vi "Initialise ctrl values.vi"(8 "error in (no error)":errorcluster) -> (0 "error out":errorcluster)   [LabVIEW 2020]
uses:
  Typedefs/HW config states enum.ctl
  Typedefs/Read Write Enum.ctl
  Typedefs/AOL modes.ctl
  Global Variables/gl_UI Ctrl Refs.vi
  Peripherals Control/Pockels/Globals/gl_Pockels control globals.vi
  Global Variables/General Globals.vi
  Typedefs/Laser control knob.ctl
  Typedefs/PMT control knob.ctl
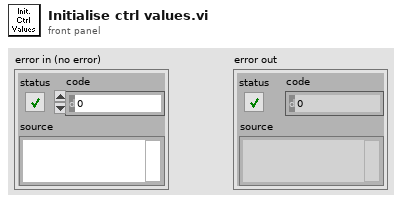
[diagram p1: front panel]
types:
  T1 = typedef "HW config states enum.ctl" = enum16{"Load from file", "Save to file", "Save backup", "Write all", "Read all", "Write XY stage settings", "Write DAQ FPGA settings", "Write Control FPGA settings", "Write Phys Channels", "Write System Config", "Write HW Config", "Save System Config", "Save HW Config", "Clear", "Compare from file"}
  T2 = typedef "UI ctrl refs cluster.ctl" = cluster{"Top level VI path":path, "Top level VI ref":refnum<vi>, "User menu ref":refnum<k9>, "Sub Panel control":refnum<vi>, "Imaging Param Tab":refnum<vi>, "Occurrence-Start drivers":refnum<k4>, "Occurrence-Speed logging initialised":refnum<k4>, "Occurrence-XYZ stage initialised":refnum<k4>, "Exit button":refnum<vi>, "Status ind":refnum<vi>, "Set as origin":refnum<vi>, "Speed Logging":refnum<vi>, "Time Lapse":refnum<vi>, "Live Imaging":refnum<vi>, "AOL Z Stack":refnum<vi>, "Motor Z Stack":refnum<vi>, "Funct Acq button":refnum<vi>, "Hard Shutter":refnum<vi>, "Virtual Shutter":refnum<vi>, "Laser Power":refnum<vi>, "AOL Mode":refnum<vi>, "Frame Size":refnum<vi>, "Field of View":refnum<vi>, "Dwell Time":refnum<vi>, "Zoom":refnum<vi>, "AOL Z":refnum<vi>, "Objective":refnum<vi>, "Axis":refnum<vi>, "Paths & Names":refnum<vi>, "Experiment folder path (ind.)":refnum<vi>, "Last State (Ind.)":refnum<vi>, "Averages":refnum<vi>, "Angle (degrees)":refnum<vi>, "X centre":refnum<vi>, "Y centre":refnum<vi>, "Plane Mode":refnum<vi>, "# Planes":refnum<vi>, "Z Start":refnum<vi>, "Z Stop":refnum<vi>, "Z Step":refnum<vi>, "PMT 1":refnum<vi>, "PMT 2":refnum<vi>, "Stage XYZ Position":refnum<vi>, "Pockels@Z Start":refnum<vi>, "Pockels@Z Stop":refnum<vi>, "Obtain Z Start":refnum<vi>, "Obtain Z Stop":refnum<vi>, "Live stim.trig.period":refnum<vi>, "Live stim.trig.enable":refnum<vi>, "Movement Correction":refnum<vi>, "Load Reference Image":refnum<vi>, "XY Stage Move":refnum<vi>, "MovCor Cluster":refnum<vi>, "RefDAQParam":refnum<vi>, "Funct. Acq. Pockels Modulation":refnum<vi>, "Ref Laser Power":refnum<vi>, "Enable Video Recording":refnum<vi>, "Video Record-Live Imaging":refnum<vi>, "Video Record-Funct acq":refnum<vi>, "Reference Source":refnum<vi>, "AOL Z-stack Chirps Ready (ind)":refnum<vi>, "Target time between mov.cor. ref triggers (ms)":refnum<vi>, "Funct. Acq. Ref frame save":refnum<vi>, "Tracking button":refnum<vi>, "Show ref plots window":refnum<vi>, "Center freq ind (nm)":refnum<vi>, "Pickup mode (ind)":refnum<vi>, "Logging queue (ind)":refnum<vi>, "Back aperture power (ind.)":refnum<vi>, "Power after objective (ind.)":refnum<vi>, "Switch user":refnum<vi>, "Ls1 Conn. Status":refnum<vi>, "Ls1Tuning Status":refnum<vi>, "Ls1 Faults":refnum<vi>, "Ls1 Connection":refnum<vi>, "Ls1 Mode":refnum<vi>, "Ls1 POWER [mW]":refnum<vi>, "Ls1Shutter":refnum<vi>, "Ls1 Wavelength":refnum<vi>, "Ls1 Note":refnum<vi>, "Ls1 Confirm Wav":refnum<vi>, "Ls1 PreChrp Prism1":refnum<vi>, "Ls1 PreChrp Prism2":refnum<vi>, "Ls1 wav top Ind":refnum<vi>, "Ls1 power top Ind":refnum<vi>, "Ls1 Pump peak Hold":refnum<vi>, "Ls1 Status Ind":refnum<vi>, "Ls1 wav cancel":refnum<vi>, "Experiment Type":refnum<vi>, "Biology Information":refnum<vi>, "Camera recording status":refnum<vi>}
  T3 = typedef "System Configuration.ctl" = cluster{"Laser wavelength (nm)":dbl, "DAQ FPGA System":T4, "Control system":T5}
  T4 = typedef "DAQ FPGA system config.ctl" = cluster{"Clock Freq (MHz) ":dbl, "Samples Wait after Trigger":u16, "AOD fill":u16, "StartupDelay":i32, "Slip Cycle (clock cycles)":u32, "Add Cycle":bool}
  T5 = typedef "CTRL system config.ctl" = cluster{"AOD 1 Amplitude":i16, "AOD 2 Amplitude":i16, "AOD 3 Amplitude":i16, "AOD 4 Amplitude":i16, "AOD 5 Amplitude":i16, "AOD 6 Amplitude":i16, "T0 (ns)":dbl, "Ta (ns)":dbl, "Data Time Interval (ns)":dbl, "Ctrl FPGA Clock (MHz)":dbl}
  T6 = typedef "AOL_Globals.ctl" = cluster{"Imaging Protocol":T7, "Number of POI":u16, "Number of Miniscans":u16, "Number of Trials":u16, "Number of Cycles ":u64, "# Averaged Frames":u16, "Laser power (%)":u8, "Pockels (V)":dbl, "Acquisition Length (sec)":dbl, "Fill time (us)":dbl, "POI Dwell time (us)":dbl, "Miniscan Dwell time per pixel (us)":dbl, "PMT 1":dbl, "PMT 2":dbl, "Back Apperture (mA)":dbl, "Frame Size":T8, "Center Frequency":dbl, "Field of View (norm)":dbl, "DwellTime (us)":dbl, "Wavelength (nm)":dbl, "Zoom":dbl, "AOL Z":dbl, "AOL Mode":T9, "GridXY":dbl, "GridZ":dbl, "TriggerPeriod (sec)":dbl, "Number of Pixels in Miniscan":u16, "Experiment folder path":path, "X centre":dbl, "Y centre":dbl, "Angle (degrees)":dbl, "Plane Mode":T10, "Threshold":u16[], "Regenerate Chirps":bool, "Rectangle ROI length (pixels)":u16, "Rectangle ROI height (pixels)":u16, "AOD fill":u16, "StartupDelay":i32, "Samples Wait after Trigger":u16, "Slip Cycle":u32, "Add Cycle":bool, "Functional Mode":T11, "Z Start":dbl, "Z Stop":dbl, "# Planes":i32, "Total Pixels":i32, "Variable Miniscan Pixels":u16[], "Use Variable Length":bool, "Use Variable Resolution":bool, "Laser power (%) at Z Start":u8, "Laser power (%) at Z Stop":u8, "Ref Z Step":i8, "Ref Dwell Time (us)":dbl, "Field of View (um)":dbl}
  T7 = typedef "Imaging Protocols enum.ctl" = enum16{"AOL Z-Stack", "Motor Z Stack", "Functional Acquisition", "Single Plane Acquisition", "Volume Acquisition", "Live Imaging", "Live Plane Imaging", "Live Volume Imaging"}
  T8 = typedef "Frame Size.ctl" = u16
  T9 = typedef "AOL modes.ctl" = enum16{"Raster", "Structural", "Pointing", "Mini Scan", "Alignment"}
  T10 = typedef "Plane Mode.ctl" = u16
  T11 = typedef "Functional Mode.ctl" = enum16{"Point", "Line", "Patch", "Plane", "Volume"}
  T12 = enum8{"Enabled", "Disabled", "Disabled and Grayed Out"}
  T13 = typedef "Laser control knob.ctl" = u16
  T14 = typedef "Read Write Enum.ctl" = enum16{"Read", "Write"}
  T15 = typedef "Ref DAQ Param.ctl" = cluster{"Full Frame Size":u16, "Ref Field of View":sgl, "Ref Zoom":i8, "Ref_dwellTime":sgl, "Ref X-pixels-per-line(Npxr)":i16, "Ref Y-lines-per-image(Npyr)":i16, "Ref Z-lines-per-image":i16, "Ignore Z lines":i16, "Ref Scan Cycles":i32, "Ref threshold XY":u16, "Ref threshold Z":u16, "Ref average XY":u16, "Ref Average  Z":u16, "Proportional_scale":fxp<+,16,2>, "Integral_scale":fxp<+/-,16,12>, "Proportional_scale Z":fxp<+,16,2>, "Integral_scale Z":fxp<+/-,16,12>, "Diff_threshold":fxp<+,16,2>, "Diff_threshold _z":fxp<+,16,2>, "Sliding Average":bool, "Ref count reset enabled":bool}
  T16 = typedef "Control algorithm.ctl" = enum16{"PID", "Kalman"}
  T17 = typedef "PMT control knob.ctl" = u16
  T18 = typedef "test_fpga_control.ctl" = cluster{"x_offset_host":fxp<+/-,16,8>, "y_offset_host":fxp<+/-,16,8>, "use host offset":bool, "Set_Ref_Centroid":bool, "OldChirpCode":bool, "use array of offsets":bool, "x_offset_host array":fxp<+/-,16,8>[], "y_offset_host array ":fxp<+/-,16,8>[], "use host offset Z":bool, "swap Z":bool, "z_offset_host ":fxp<+/-,16,8>}
  T19 = typedef "Hardware Configuration settings.ctl" = cluster{"Dev. PC":bool, "Swap XY on stage":bool, "No of AOD":u8, "MC Supported":bool, "Axial MC":bool, "Computer MAC address":string, "Externalise Triggers":bool, "Trigger HW config":T20, "DAQmx Chan":T21, "XY stage available":bool, "XY Stage":T22, "Z stage available":bool, "Z Stage config cluster":T23, "Encoder available":bool, "Encoder":T24, "VidRec available":bool, "Cam VidRec":T25, "Laser Power Control HW config":T26, "Laser 1 available":bool, "Laser 1 config cluster":T27, "Prechirper 1 available":bool, "Prechirper 1 config cluster":T28, "Control system.FPGA available?":bool, "Control Sys. HW config":T29, "DAQ FPGA HW Config":T30, "PMT Voltage Range":T34}
  T20 = typedef "Triggers HW config.ctl" = cluster{"Available Device List":i32, "Device Address":string}
  T21 = typedef "DAQmx physical channels cluster.ctl" = cluster{"Pockels AO":tag, "Hard shutter AO":tag, "PMT AOs":tag, "Galvo AOs":tag, "Power meter AI":tag}
  T22 = typedef "XY Stage config cluster.ctl" = cluster{"COM port":refnum<visa-resource-name>, "Baudrate":i32, "Type":string}
  T23 = typedef "Z Stage config cluster.ctl" = cluster{"COM port":refnum<visa-resource-name>, "Baudrate":i32, "Type":string}
  T24 = typedef "Encoder config cluster.ctl" = cluster{"IP address":string, "Port":u16, "Wheel radius (cm)":dbl, "Encoder Trigger":tag}
  T25 = typedef "Cam VidRec HW config setup cluster.ctl" = cluster{"DO flag-Video record":tag, "DO flag-Trial start":tag}
  T26 = typedef "Laser Power Control HW config.ctl" = cluster{"Laser Power Control":string, "Laser Power Modulation Control":enum16{"NI", "FPGA"}}
  T27 = typedef "Laser 1 config cluster.ctl" = cluster{"COM port":refnum<visa-resource-name>, "Baud Rate":i32, "Type":string}
  T28 = typedef "PreChirper 1 config cluster.ctl" = cluster{"Type":string, "Baud Rate":i32, "COM port":refnum<visa-resource-name>}
  T29 = typedef "Control Sys HW config cluster.ctl" = cluster{"Control system.FPGA Type":enum16{"Virtex 5", "Virtex 7"}, "Control system.Network adapter name":string, "Control system.MAC address":string, "Control system.Ethernet Port":u32, "Control system.Ethernet Port Opened":bool}
  T30 = typedef "DAQ FPGA HW config cluster.ctl" = cluster{"FGPA Ref":T31, "Target":T32, "input card type":T33}
  T31 = typedef "FPGA Ref.ctl" = refnum<k20>
  T32 = typedef "nirio_resource_hc.ctl" = tag
  T33 = typedef "FPGA input type AC-DC.ctl" = enum16{"AC Card", "DC Card"}
  T34 = typedef "PMT Voltage Range.ctl" = cluster{"PMT Voltage Lower Limit":dbl, "PMT Voltage Upper Limit":dbl}
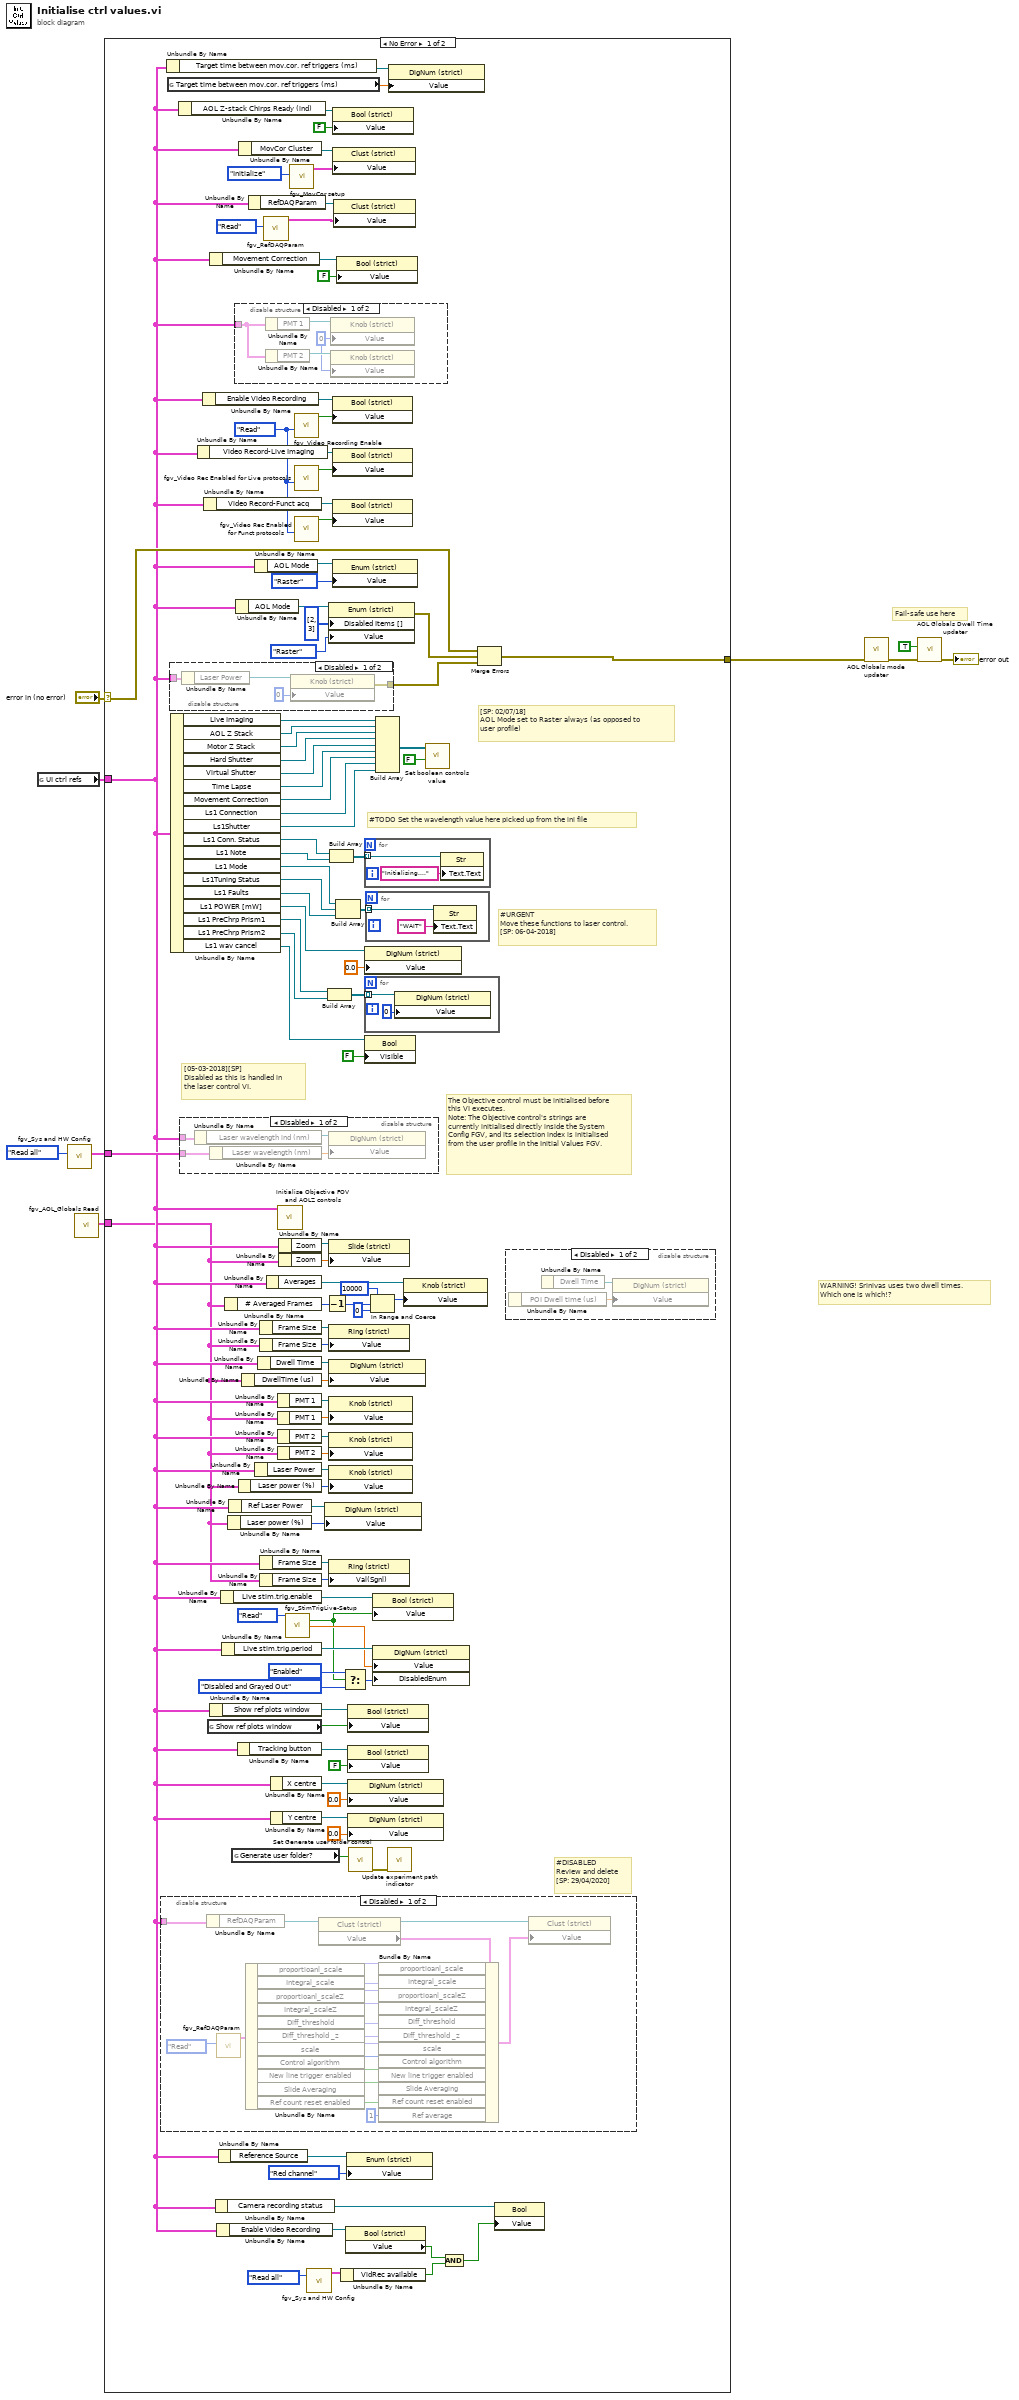
[diagram p0: block diagram]
diagram:
  # "Fail-safe use here"
  # "WARNING! Srinivas uses two dwell times.\nWhich one is which!?"
  n1 = global read "gl_UI Ctrl Refs.vi" "UI ctrl refs"() -> (w8:T2)
  n2 = call "fgv_Sys and HW Config.vi"("Function"=HW_config_states_enum."Read all") -> ("System Config OUT"=w1:T3)  [unwired: 8 in, 2 out]
  n3 = call "fgv_AOL_Globals Read.vi"() -> ("AOL_Globals"=w6:T6)  [unwired: 9 in, 2 out]
  n4 = case shown="No Error" "error in (no error)" {
    selector: "error in (no error)" -> [w45 w154]
    tunnel: w8 -> [w11 _]
    tunnel: [w102 w154] -> w5
    tunnel: w6 -> [w10 _]
    tunnel: w1 -> [w53 _]
    frame No Error {
      w96 = Read_Write_Enum."Read" ("Function")
      # "#DISABLED\nReview and delete\n[SP: 29/04/2020]"
      # "[SP: 02/07/18]\nAOL Mode set to Raster always (as opposed to \nuser profile)"
      # "#URGENT \nMove these functions to laser control.\n[SP: 06-04-2018]"
      # "[05-03-2018][SP]\nDisabled as this is handled in \nthe laser control VI."
      # "#TODO Set the wavelength value here picked up from the ini file"
      # "The Objective control must be initialised before this VI executes.\nNote: The Objective control's strings are currently initialised directly inside the System Config FGV, and its selection index is initialised from the user profile in the Initial Values FGV."
      n5 = disable-structure shown="Disabled" {
        disable-tunnel: w11 -> [w115 _]
        frame Disabled {
          n6 = Unbundle By Name(w115) -> ("RefDAQParam"=w133:refnum<vi>)
          n7 = call "fgv_RefDAQParam.vi"("Function"=enum16{"Initialize", "Write", "Read"}."Read") -> ("RefDAQParam"=w129:T15)  [unwired: 9 in, 1 out]
          n8 = Unbundle By Name(w129) -> ("proportioanl_scale"=w128:fxp<+,16,2>, "Integral_scale"=w127:fxp<+/-,16,12>, "proportioanl_scaleZ"=w126:fxp<+,16,2>, "Integral_scaleZ"=w125:fxp<+/-,16,12>, "Diff_threshold"=w124:fxp<+,16,2>, "Diff_threshold _z"=w123:fxp<+,16,2>, "scale"=w122:fxp<+,16,2>, "Control algorithm"=w121:T16, "New line trigger enabled"=w120:bool, "Slide Averaging"=w119:bool, "Ref count reset enabled"=w118:bool)
          n9 = property class="Clust (strict)"(reference=w133) -> (reference out=w117:refnum<vi>, "Value"=w132:T15)  [unwired: 1 in, 1 out]
          n10 = Bundle By Name(cluster=w132, "proportioanl_scale"=w128, "Integral_scale"=w127, "proportioanl_scaleZ"=w126, "Integral_scaleZ"=w125, "Diff_threshold"=w124, "Diff_threshold _z"=w123, "scale"=w122, "Control algorithm"=w121, "New line trigger enabled"=w120, "Slide Averaging"=w119, "Ref count reset enabled"=w118, "Ref average"=u16 1) -> (w131:T15)
          n11 = property class="Clust (strict)"(reference=w117, "Value"=w131) -> ()  [unwired: 1 in, 2 out]
        }
        frame Enabled {
        }
      }
      n12 = Unbundle By Name(w11) -> ("Target time between mov.cor. ref triggers (ms)"=w83:refnum<vi>)
      n13 = global read "gl_Pockels control globals.vi" "Target time between mov.cor. ref triggers (ms)"() -> (w82:dbl)
      n14 = disable-structure shown="Disabled" {
        disable-tunnel: [w147 _] -> w103
        disable-tunnel: w11 -> [w146 _]
        frame Disabled {
          n15 = Unbundle By Name(w146) -> ("Laser Power"=w149:refnum<vi>)
          n16 = property class="Knob (strict)"(reference=w149, "Value"=T13 0) -> (error out=w147:errorcluster)  [unwired: 1 in, 1 out]
        }
        frame Enabled {
        }
      }
      n17 = Unbundle By Name(w11) -> ("Live Imaging"=w114:refnum<vi>, "AOL Z Stack"=w113:refnum<vi>, "Motor Z Stack"=w112:refnum<vi>, "Hard Shutter"=w111:refnum<vi>, "Virtual Shutter"=w110:refnum<vi>, "Time Lapse"=w107:refnum<vi>, "Movement Correction"=w101:refnum<vi>, "Ls1 Connection"=w43:refnum<vi>, "Ls1Shutter"=w42:refnum<vi>, "Ls1 Conn. Status"=w41:refnum<vi>, "Ls1 Note"=w40:refnum<vi>, "Ls1 Mode"=w37:refnum<vi>, "Ls1Tuning Status"=w36:refnum<vi>, "Ls1 Faults"=w35:refnum<vi>, "Ls1 POWER [mW]"=w34:refnum<vi>, "Ls1 PreChrp Prism1"=w32:refnum<vi>, "Ls1 PreChrp Prism2"=w31:refnum<vi>, "Ls1 wav cancel"=w28:refnum<vi>)
      n18 = Unbundle By Name(w11) -> ("AOL Z-stack Chirps Ready (ind)"=w85:refnum<vi>)
      n19 = disable-structure shown="Disabled" {
        disable-tunnel: w53 -> [w135 _]
        disable-tunnel: w11 -> [w134 _]
        frame Disabled {
          n20 = Unbundle By Name(w134) -> ("Laser wavelength ind (nm)"=w137:refnum<vi>)
          n21 = Unbundle By Name(w135) -> ("Laser wavelength (nm)"=w136:dbl)
          n22 = property on="Property Node" class="DigNum (strict)"(reference=w137, "Value"=w136) -> ()  [unwired: 1 in, 2 out]
        }
        frame Enabled {
        }
      }
      n23 = Unbundle By Name(w11) -> ("Video Record-Live Imaging"=w95:refnum<vi>)
      n24 = Unbundle By Name(w11) -> ("Enable Video Recording"=w98:refnum<vi>)
      n25 = Unbundle By Name(w11) -> ("Video Record-Funct acq"=w94:refnum<vi>)
      n26 = global read "General Globals.vi" "Show ref plots window"() -> (w54:bool)
      n27 = Unbundle By Name(w11) -> ("Movement Correction"=w22:refnum<vi>)
      n28 = Unbundle By Name(w11) -> ("Show ref plots window"=w55:refnum<vi>)
      n29 = Unbundle By Name(w11) -> ("Camera recording status"=w15:refnum<vi>)
      n30 = Unbundle By Name(w11) -> ("Enable Video Recording"=w19:refnum<vi>)
      n31 = Unbundle By Name(w11) -> ("Reference Source"=w24:refnum<vi>)
      n32 = Unbundle By Name(w11) -> ("Live stim.trig.enable"=w62:refnum<vi>)
      n33 = Unbundle By Name(w11) -> ("Live stim.trig.period"=w61:refnum<vi>)
      n34 = Unbundle By Name(w10) -> ("# Averaged Frames"=w79:u16)
      n35 = Unbundle By Name(w10) -> ("Laser power (%)"=w13:u8)
      n36 = Unbundle By Name(w11) -> ("Ref Laser Power"=w12:refnum<vi>)
      n37 = global read "General Globals.vi" "Generate user folder?"() -> (w44:bool)
      n38 = disable-structure shown="Disabled" {
        disable-tunnel: w11 -> [w151 _]
        frame Disabled {
          w150 = T17 0 ("Value")
          n39 = Unbundle By Name(w151) -> ("PMT 1"=w153:refnum<vi>)
          n40 = Unbundle By Name(w151) -> ("PMT 2"=w152:refnum<vi>)
          n41 = property on="Property Node" class="Knob (strict)"(reference=w153, "Value"=w150) -> ()  [unwired: 1 in, 2 out]
          n42 = property on="Property Node" class="Knob (strict)"(reference=w152, "Value"=w150) -> ()  [unwired: 1 in, 2 out]
        }
        frame Enabled {
        }
      }
      n43 = Unbundle By Name(w11) -> ("AOL Mode"=w105:refnum<vi>)
      n44 = Unbundle By Name(w11) -> ("Tracking button"=w52:refnum<vi>)
      n45 = Unbundle By Name(w10) -> ("Laser power (%)"=w64:u8)
      n46 = Unbundle By Name(w11) -> ("MovCor Cluster"=w86:refnum<vi>)
      n47 = Unbundle By Name(w10) -> ("DwellTime (us)"=w70:dbl)
      n48 = Unbundle By Name(w11) -> ("RefDAQParam"=w89:refnum<vi>)
      n49 = Unbundle By Name(w11) -> ("AOL Mode"=w100:refnum<vi>)
      n50 = Unbundle By Name(w11) -> ("Laser Power"=w65:refnum<vi>)
      n51 = Unbundle By Name(w11) -> ("Dwell Time"=w71:refnum<vi>)
      n52 = Unbundle By Name(w11) -> ("Frame Size"=w72:refnum<vi>)
      n53 = Unbundle By Name(w10) -> ("Frame Size"=w73:T8)
      n54 = Unbundle By Name(w11) -> ("Frame Size"=w91:refnum<vi>)
      n55 = Unbundle By Name(w10) -> ("Frame Size"=w63:T8)
      n56 = call "fgv_RefDAQParam.vi"("Function"=enum16{"Initialize", "Write", "Read"}."Read" ("Status")) -> ("RefDAQParam"=w90:T15)  [unwired: 9 in, 1 out]
      n57 = Unbundle By Name(w11) -> ("Averages"=w78:refnum<vi>)
      n58 = Unbundle By Name(w11) -> ("X centre"=w50:refnum<vi>)
      n59 = Unbundle By Name(w11) -> ("Y centre"=w49:refnum<vi>)
      n60 = Unbundle By Name(w11) -> ("PMT 1"=w68:refnum<vi>)
      n61 = Unbundle By Name(w10) -> ("PMT 1"=w67:dbl)
      n62 = Unbundle By Name(w11) -> ("PMT 2"=w69:refnum<vi>)
      n63 = Unbundle By Name(w10) -> ("PMT 2"=w66:dbl)
      n64 = call "Initialise Objective FOV and AOLZ controls.vi"("UI ctrl refs"=w11) -> ()  [unwired: 10 in, 1 out]
      n65 = Unbundle By Name(w11) -> ("Zoom"=w81:refnum<vi>)
      n66 = Unbundle By Name(w10) -> ("Zoom"=w80:dbl)
      n67 = call "fgv_StimTrigLive-Setup.vi"("Function"=enum16{"Intialize", "Write", "Read", "Clear"}."Read") -> ("Live stim.trig.enable"=w46:bool, "Live stim.trig.period (sec)"=w59:dbl)  [unwired: 11 in, 2 out]
      n68 = call "fgv_MovCor setup.vi"("Status"=enum16{"Initialize", "Write", "Read"}."Initialize") -> ("MovCor Cluster"=w29:T18)  [unwired: 9 in, 1 out]
      n69 = call "fgv_Video Recording Enable.vi"("Function"=w96) -> ("Video Recording Enabled"=w97:bool)  [unwired: 9 in, 1 out]
      n70 = call "fgv_Video Rec Enabled for Live protocols.vi"("Function"=w96) -> ("Video Recording Enabled for Live protocols"=w92:bool)  [unwired: 10 in]
      n71 = call "fgv_Video Rec Enabled for Funct protocols.vi"("Function"=w96) -> ("Video Recording Enabled for functional acq protocols"=w93:bool)  [unwired: 10 in]
      n72 = call "fgv_Sys and HW Config.vi"("Function"=HW_config_states_enum."Read all") -> ("Hardware Configuration OUT"=w18:T19)  [unwired: 8 in, 2 out]
      n73 = Decrement(x=w79) -> (x-1=w77:u16)
      n74 = property class="DigNum (strict)"(reference=w12, "Value"=w13) -> ()  [unwired: 1 in, 2 out]
      n75 = Build Array(w32, w31) -> (w30:refnum<vi>[])
      n76 = property on="Property Node" class="Enum (strict)"(reference=w105, "Disabled Items []"=i32[] [2, 3], "Value"=AOL_modes."Raster") -> (error out=w104:errorcluster)  [unwired: 1 in, 1 out]
      n77 = property on="Property Node" class="Slide (strict)"(reference=w81, "Value"=w80) -> ()  [unwired: 1 in, 2 out]
      n78 = property on="Property Node" class="Ring (strict)"(reference=w72, "Value"=w73) -> ()  [unwired: 1 in, 2 out]
      n79 = property on="Property Node" class="DigNum (strict)"(reference=w71, "Value"=w70) -> ()  [unwired: 1 in, 2 out]
      n80 = property class="Knob (strict)"(reference=w68, "Value"=w67) -> ()  [unwired: 1 in, 2 out]
      n81 = property class="Knob (strict)"(reference=w69, "Value"=w66) -> ()  [unwired: 1 in, 2 out]
      n82 = property class="Knob (strict)"(reference=w65, "Value"=w64) -> ()  [unwired: 1 in, 2 out]
      n83 = property on="Property Node" class="Ring (strict)"(reference=w91, "Val(Sgnl)"=w63) -> ()  [unwired: 1 in, 2 out]
      n84 = Build Array(w41, w40) -> (w39:refnum<vi>[])
      n85 = property on="Property Node" class="Bool (strict)"(reference=w98, "Value"=w97) -> ()  [unwired: 1 in, 2 out]
      n86 = property on="Property Node" class="Bool (strict)"(reference=w95, "Value"=w92) -> ()  [unwired: 1 in, 2 out]
      n87 = property on="Property Node" class="Bool (strict)"(reference=w94, "Value"=w93) -> ()  [unwired: 1 in, 2 out]
      n88 = property on="Property Node" class="Enum (strict)"(reference=w100, "Value"=AOL_modes."Raster") -> ()  [unwired: 1 in, 2 out]
      n89 = property class="Bool (strict)"(reference=w85, "Value"=FALSE) -> ()  [unwired: 1 in, 2 out]
      n90 = property class="Clust (strict)"(reference=w86, "Value"=w29) -> ()  [unwired: 1 in, 2 out]
      n91 = property class="Clust (strict)"(reference=w89, "Value"=w90) -> ()  [unwired: 1 in, 2 out]
      n92 = Build Array(w37, w36, w35) -> (w38:refnum<vi>[])
      n93 = property class="Bool (strict)"(reference=w22, "Value"=FALSE) -> ()  [unwired: 1 in, 2 out]
      n94 = Unbundle By Name(w18) -> ("VidRec available"=w16:bool)
      n95 = Select(t=T12."Enabled" ("Disabled"), s=w46, f=T12."Disabled and Grayed Out" ("Disabled")) -> (s? t:f=w58:T12)
      n96 = property class="Bool (strict)"(reference=w19) -> ("Value"=w17:bool)  [unwired: 1 in, 2 out]
      n97 = property class="Enum (strict)"(reference=w24, "Value"=enum16{"Green channel", "Red channel"}."Red channel") -> ()  [unwired: 1 in, 2 out]
      n98 = property on="Property Node" class="Bool (strict)"(reference=w55, "Value"=w54) -> ()  [unwired: 1 in, 2 out]
      n99 = property on="Property Node" class="Bool (strict)"(reference=w52, "Value"=FALSE) -> ()  [unwired: 1 in, 2 out]
      n100 = property class="DigNum (strict)"(reference=w50, "Value"=0.0) -> ()  [unwired: 1 in, 2 out]
      n101 = property class="DigNum (strict)"(reference=w49, "Value"=0.0) -> ()  [unwired: 1 in, 2 out]
      n102 = call "Set Generate user folder control.vi"("Generate user folder?"=w44) -> ("error out"=w25:errorcluster)  [unwired: 10 in]
      n103 = for {
        tunnel: w39 -> [w143] mode=indexing
        n104 = property class="Str"(reference=w143, "Text.Text"="Initialising....") -> ()  [unwired: 1 in, 2 out]
      }
      n105 = property class="Bool"(reference=w28, "Visible"=FALSE) -> ()  [unwired: 1 in, 2 out]
      n106 = property class="DigNum (strict)"(reference=w34, "Value"=0.0) -> ()  [unwired: 1 in, 2 out]
      n107 = for {
        tunnel: w30 -> [w139] mode=indexing
        n108 = property class="DigNum (strict)"(reference=w139, "Value"=0) -> ()  [unwired: 1 in, 2 out]
      }
      n109 = for {
        tunnel: w38 -> [w141] mode=indexing
        n110 = property class="Str"(reference=w141, "Text.Text"="WAIT") -> ()  [unwired: 1 in, 2 out]
      }
      n111 = In Range and Coerce(upper limit=u16 10000, x=w77, lower limit=u16 0) -> (coerced(x)=w76:u16)  [unwired: 1 out]
      n112 = property on="Property Node" class="Bool (strict)"(reference=w62, "Value"=w46) -> ()  [unwired: 1 in, 2 out]
      n113 = property on="Property Node" class="DigNum (strict)"(reference=w61, "Value"=w59, "DisabledEnum"=w58) -> ()  [unwired: 1 in, 2 out]
      n114 = Build Array(w114, w113, w112, w111, w110, w107, w101, w43, w42) -> (w109:refnum<vi>[])
      n115 = call "Update experiment path indicator.vi"("error in (no error)"=w25) -> ()  [unwired: 9 in, 2 out]
      n116 = property class="DigNum (strict)"(reference=w83, "Value"=w82) -> ()  [unwired: 1 in, 2 out]
      n117 = property on="Property Node" class="Knob (strict)"(reference=w78, "Value"=w76) -> ()  [unwired: 1 in, 2 out]
      n118 = call "Set boolean controls value.vi"("Value"=FALSE, "Boolean ctrl ref array"=w109) -> ()  [unwired: 10 in]
      n119 = And(x=w17, y=w16) -> (x .and. y?=w14:bool)
      n120 = Merge Errors(w45, w104, w103) -> (w102:errorcluster)
      n121 = property class="Bool"(reference=w15, "Value"=w14) -> ()  [unwired: 1 in, 2 out]
      n122 = disable-structure shown="Disabled" {
        frame Disabled {
          n123 = Unbundle By Name() -> ("POI Dwell time (us)"=w145:dbl)  [unwired: 1 in]
          n124 = Unbundle By Name() -> ("Dwell Time"=w144:refnum<vi>)  [unwired: 1 in]
          n125 = property on="Property Node" class="DigNum (strict)"(reference=w144, "Value"=w145) -> ()  [unwired: 1 in, 2 out]
        }
        frame Enabled {
        }
      }
    }
    frame Error {
    }
  }
  n126 = call "AOL Globals mode updater.vi"("error in"=w5) -> ("error out"=w4:errorcluster)  [unwired: 10 in]
  n127 = call "AOL Globals Dwell Time updater.vi"("error in"=w4, "Disable message (F)"=TRUE) -> ("error out"=→"error out":errorcluster)  [unwired: 9 in]
